vi "BRig_RT__Case_Exp__State_WrongOrTimeout_Pre.vi"(6 "input_dataExp":u16[](array[numeric]), 8 "input_dataTrial":u16[][](array[numeric]), 9 "input_dataBlock":u16[][](array[numeric]), 10 "input_WorTO":bool, 11 "input_dataCurrent":u16[](array[numeric])) -> (0 "output_dataTrial":u16[][](array[numeric]), 1 "output_dataBlock":u16[][](array[numeric]), 2 "output_T2R_or_BTPR":u16, 3 "output_dataCurrent":u16[](array[numeric]), 5 "output_T2R":bool, 7 "output_BTPR":bool)   [LabVIEW 2014]
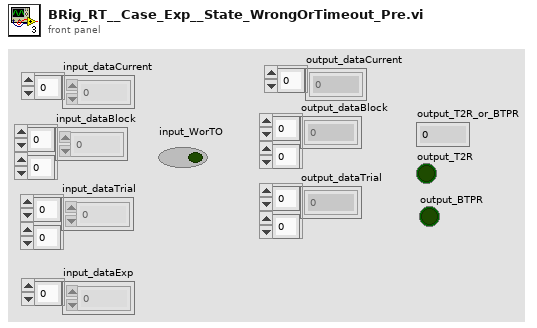
[diagram p1: front panel]
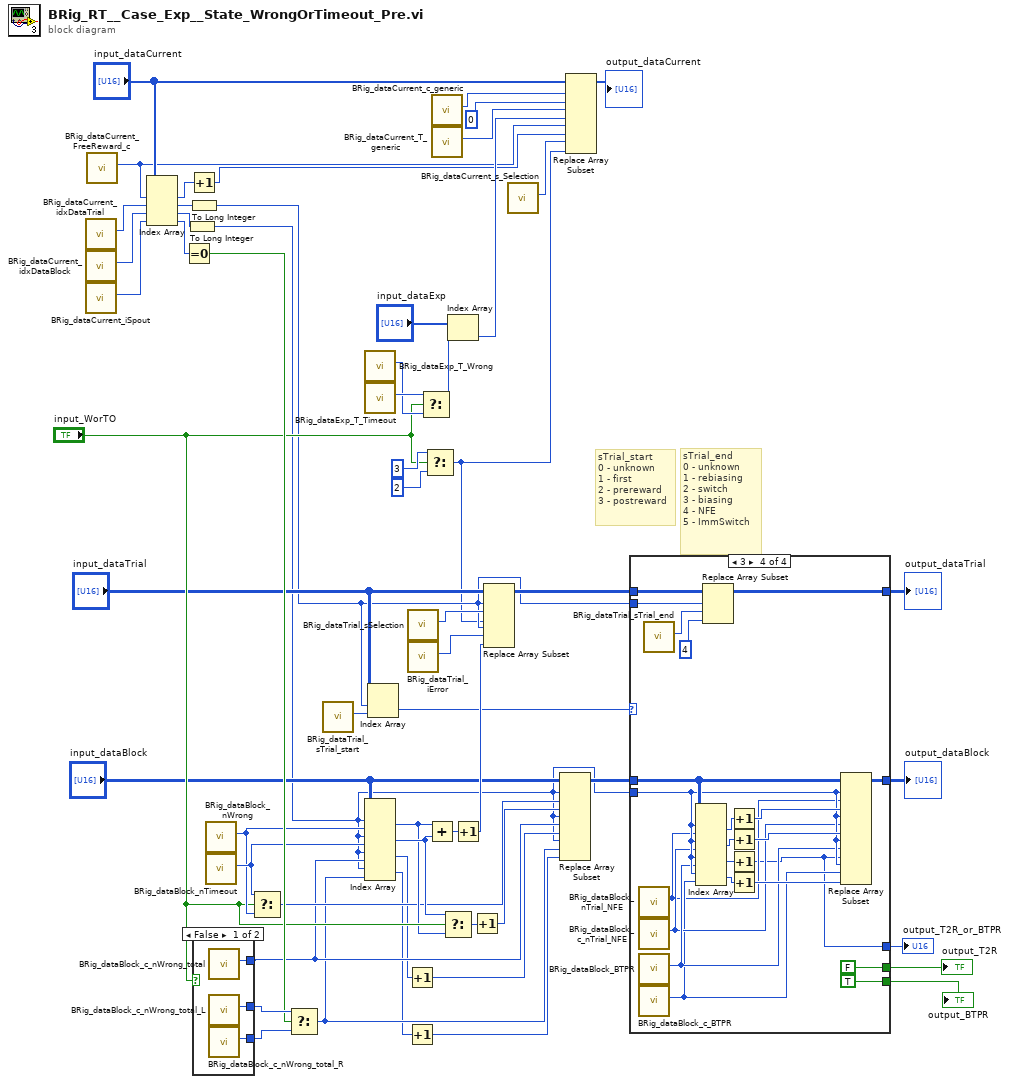
[diagram p0: block diagram]
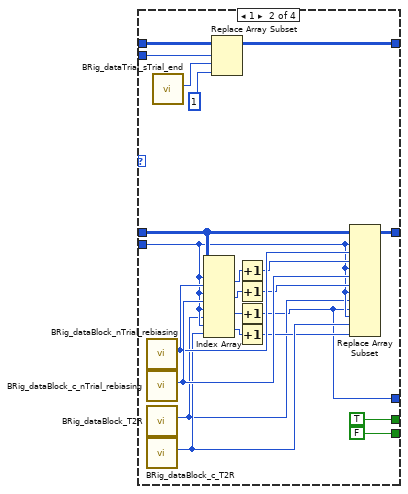
[diagram p3: hidden frame]
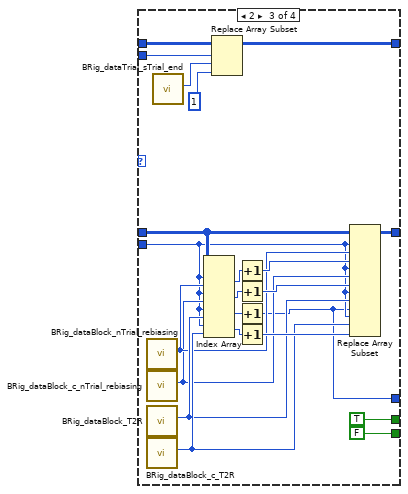
[diagram p4: hidden frame]
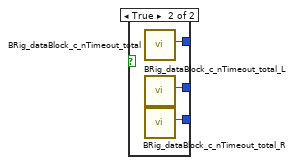
[diagram p5: hidden frame]
diagram:
  # "sTrial_end\n0 - unknown\n1 - rebiasing\n2 - switch\n3 - biasing\n4 - NFE\n5 - ImmSwitch"
  # "sTrial_start\n0 - unknown\n1 - first\n2 - prereward\n3 - postreward"
  n1 = call "BRig_dataCurrent_idxDataTrial.vi"() -> ("output_idxDataTrial"=w53:i32)  [unwired: 11 in]
  n2 = call "BRig_dataCurrent_idxDataBlock.vi"() -> ("output_idxDataBlock"=w51:i32)  [unwired: 11 in]
  n3 = call "BRig_dataCurrent_iSpout.vi"() -> ("output_iSpout"=w49:i32)  [unwired: 11 in]
  n4 = call "BRig_dataCurrent_FreeReward_c.vi"() -> ("output_FreeReward_c"=w8:i32)  [unwired: 11 in]
  n5 = Index Array(array="input_dataCurrent", index #1=w8, index #2=w53, index #3=w51, index #4=w49) -> (element #1=w9:u16, element #2=w52:u16, element #3=w50:u16, element #4=w48:u16)
  n6 = Equal To 0?(x=w48) -> (x = 0?=w33:bool)
  n7 = To Long Integer(number=w50) -> (32bit integer=w13:i32)
  n8 = Increment(x=w9) -> (x+1=w7:u16)
  n9 = To Long Integer(number=w52) -> (32bit integer=w5:i32)
  n10 = case shown="False" "input_WorTO" {
    tunnel: [w60 w63] -> w23
    tunnel: [w59 w62] -> w37
    tunnel: [w58 w61] -> w36
    frame False {
      n11 = call "BRig_dataBlock_c_nWrong_total.vi"() -> ("output_c_nWrong_total"=w60:i32)  [unwired: 11 in]
      n12 = call "BRig_dataBlock_c_nWrong_total_L.vi"() -> ("output_c_nWrong_total_L"=w59:i32)  [unwired: 11 in]
      n13 = call "BRig_dataBlock_c_nWrong_total_R.vi"() -> ("output_c_nWrong_total_R"=w58:i32)  [unwired: 11 in]
    }
    frame True {
      n14 = call "BRig_dataBlock_c_nTimeout_total.vi"() -> ("output_c_nTimeout_total"=w63:i32)  [unwired: 11 in]
      n15 = call "BRig_dataBlock_c_nTimeout_total_L.vi"() -> ("output_c_nTimeout_total_L"=w62:i32)  [unwired: 11 in]
      n16 = call "BRig_dataBlock_c_nTimeout_total_R.vi"() -> ("output_c_nTimeout_total_R"=w61:i32)  [unwired: 11 in]
    }
  }
  n17 = call "BRig_dataBlock_nWrong.vi"() -> ("output_nWrong"=w31:i32)  [unwired: 11 in]
  n18 = call "BRig_dataBlock_nTimeout.vi"() -> ("output_nTimeout"=w32:i32)  [unwired: 11 in]
  n19 = Select(t=w32, s="input_WorTO", f=w31) -> (s? t:f=w25:i32)
  n20 = Select(t=w37, s=w33, f=w36) -> (s? t:f=w22:i32)
  n21 = call "BRig_dataTrial_sTrial_start.vi"() -> ("output_sTrial_start"=w17:i32)  [unwired: 11 in]
  n22 = call "BRig_dataExp_T_Wrong.vi"() -> ("output_T_Wrong"=w43:i32)  [unwired: 11 in]
  n23 = call "BRig_dataExp_T_Timeout.vi"() -> ("output_T_Timeout"=w44:i32)  [unwired: 11 in]
  n24 = Index Array(array="input_dataBlock", index (row) #1=w13, index (col) #1=w31, index (row) #2=w13, index (col) #2=w32, index (row) #3=w13, index (col) #3=w23, index (row) #4=w13, index (col) #4=w22) -> (element #1=w28:u16, element #2=w29:u16, element #3=w21:u16, element #4=w20:u16)
  n25 = Index Array(array="input_dataTrial", index (row)=w5, index (col)=w17) -> (element=w12:u16)
  n26 = Increment(x=w21) -> (x+1=w19:u16)
  n27 = Increment(x=w20) -> (x+1=w18:u16)
  n28 = call "BRig_dataTrial_sSelection.vi"() -> ("output_sSelection"=w39:i32)  [unwired: 11 in]
  n29 = call "BRig_dataTrial_iError.vi"() -> ("output_iError"=w38:i32)  [unwired: 11 in]
  n30 = Select(t=w44, s="input_WorTO", f=w43) -> (s? t:f=w45:i32)
  n31 = Select(t=u16 3 ("new element/subarray"), s="input_WorTO", f=u16 2 ("new element/subarray")) -> (s? t:f=w4:u16)
  n32 = Add(x=w28, y=w29) -> (x+y=w35:u16)
  n33 = call "BRig_dataCurrent_c_generic.vi"() -> ("output_count_generic"=w56:i32)  [unwired: 11 in]
  n34 = call "BRig_dataCurrent_T_generic.vi"() -> ("output_T_generic"=w55:i32)  [unwired: 11 in]
  n35 = Select(t=w29, s="input_WorTO", f=w28) -> (s? t:f=w27:u16)
  n36 = Index Array(array="input_dataExp", index=w45) -> (element=w42:u16)
  n37 = Increment(x=w35) -> (x+1=w34:u16)
  n38 = Increment(x=w27) -> (x+1=w24:u16)
  n39 = Replace Array Subset(array="input_dataTrial", new element #1=w4, index (row) #1=w5, index (col) #1=w39, new element #2=w34, index (row) #2=w5, index (col) #2=w38) -> (w15:u16[][])
  n40 = call "BRig_dataCurrent_s_Selection.vi"() -> ("output_s_Selection"=w6:i32)  [unwired: 11 in]
  n41 = Replace Array Subset(array="input_dataBlock", new element #1=w24, index (row) #1=w13, index (col) #1=w25, new element #2=w19, index (row) #2=w13, index (col) #2=w23, new element #3=w18, index (row) #3=w13, index (col) #3=w22) -> (w14:u16[][])
  n42 = Replace Array Subset(array="input_dataCurrent", new element #1=u16 0 ("new element/subarray"), index #1=w56, new element #2=w42, index #2=w55, new element #3=w7, index #3=w8, new element #4=w4, index #4=w6) -> (→"output_dataCurrent":u16[])
  n43 = case shown="3" w12 {
    tunnel: w15 -> [w65 w87 w109 w131]
    tunnel: w5 -> [_ w85 w107 w129]
    tunnel: [w65 w86 w108 w130] -> w10
    tunnel: w14 -> [w64 w76 w93 w119]
    tunnel: [w64 w75 w91 w117] -> w11
    tunnel: w13 -> [_ w72 w92 w118]
    tunnel: [_ w66 w90 w110] -> w3
    tunnel: [_ TRUE TRUE FALSE] -> w2
    tunnel: [_ FALSE FALSE TRUE] -> w1
    frame 0, Default {
    }
    frame 1 {
      n44 = call "BRig_dataBlock_nTrial_rebiasing.vi"() -> ("output_nTrial_rebiasing"=w81:i32)  [unwired: 11 in]
      n45 = call "BRig_dataBlock_c_nTrial_rebiasing.vi"() -> ("output_c_nTrial_rebiasing"=w82:i32)  [unwired: 11 in]
      n46 = call "BRig_dataBlock_T2R.vi"() -> ("output_T2R"=w69:i32)  [unwired: 11 in]
      n47 = call "BRig_dataBlock_c_T2R.vi"() -> ("output_c_T2R"=w71:i32)  [unwired: 11 in]
      n48 = call "BRig_dataTrial_sTrial_end.vi"() -> ("output_sTrial_end"=w84:i32)  [unwired: 11 in]
      n49 = Index Array(array=w76, index (row) #1=w72, index (col) #1=w81, index (row) #2=w72, index (col) #2=w82, index (row) #3=w72, index (col) #3=w69, index (row) #4=w72, index (col) #4=w71) -> (element #1=w80:u16, element #2=w78:u16, element #3=w74:u16, element #4=w73:u16)
      n50 = Replace Array Subset(array=w87, new element=u16 1 ("new element/subarray"), index (row)=w85, index (col)=w84) -> (w86:u16[][])
      n51 = Increment(x=w80) -> (x+1=w79:u16)
      n52 = Increment(x=w78) -> (x+1=w77:u16)
      n53 = Increment(x=w74) -> (x+1=w66:u16)
      n54 = Increment(x=w73) -> (x+1=w70:u16)
      n55 = Replace Array Subset(array=w76, new element #1=w79, index (row) #1=w72, index (col) #1=w81, new element #2=w77, index (row) #2=w72, index (col) #2=w82, new element #3=w66, index (row) #3=w72, index (col) #3=w69, new element #4=w70, index (row) #4=w72, index (col) #4=w71) -> (w75:u16[][])
    }
    frame 2 {
      n56 = call "BRig_dataBlock_nTrial_rebiasing.vi"() -> ("output_nTrial_rebiasing"=w95:i32)  [unwired: 11 in]
      n57 = call "BRig_dataBlock_c_nTrial_rebiasing.vi"() -> ("output_c_nTrial_rebiasing"=w94:i32)  [unwired: 11 in]
      n58 = call "BRig_dataBlock_T2R.vi"() -> ("output_T2R"=w102:i32)  [unwired: 11 in]
      n59 = call "BRig_dataBlock_c_T2R.vi"() -> ("output_c_T2R"=w103:i32)  [unwired: 11 in]
      n60 = call "BRig_dataTrial_sTrial_end.vi"() -> ("output_sTrial_end"=w106:i32)  [unwired: 11 in]
      n61 = Index Array(array=w93, index (row) #1=w92, index (col) #1=w95, index (row) #2=w92, index (col) #2=w94, index (row) #3=w92, index (col) #3=w102, index (row) #4=w92, index (col) #4=w103) -> (element #1=w96:u16, element #2=w98:u16, element #3=w100:u16, element #4=w101:u16)
      n62 = Replace Array Subset(array=w109, new element=u16 1 ("new element/subarray"), index (row)=w107, index (col)=w106) -> (w108:u16[][])
      n63 = Increment(x=w96) -> (x+1=w97:u16)
      n64 = Increment(x=w98) -> (x+1=w99:u16)
      n65 = Increment(x=w100) -> (x+1=w90:u16)
      n66 = Increment(x=w101) -> (x+1=w104:u16)
      n67 = Replace Array Subset(array=w93, new element #1=w97, index (row) #1=w92, index (col) #1=w95, new element #2=w99, index (row) #2=w92, index (col) #2=w94, new element #3=w90, index (row) #3=w92, index (col) #3=w102, new element #4=w104, index (row) #4=w92, index (col) #4=w103) -> (w91:u16[][])
    }
    frame 3 {
      n68 = call "BRig_dataBlock_nTrial_NFE.vi"() -> ("output_nTrial_NFE"=w113:i32)  [unwired: 11 in]
      n69 = call "BRig_dataBlock_c_nTrial_NFE.vi"() -> ("output_c_nTrial_NFE"=w115:i32)  [unwired: 11 in]
      n70 = call "BRig_dataBlock_BTPR.vi"() -> ("output_BTPR"=w116:i32)  [unwired: 11 in]
      n71 = call "BRig_dataBlock_c_BTPR.vi"() -> ("output_c_BTPR"=w114:i32)  [unwired: 11 in]
      n72 = call "BRig_dataTrial_sTrial_end.vi"() -> ("output_sTrial_end"=w128:i32)  [unwired: 11 in]
      n73 = Index Array(array=w119, index (row) #1=w118, index (col) #1=w113, index (row) #2=w118, index (col) #2=w115, index (row) #3=w118, index (col) #3=w116, index (row) #4=w118, index (col) #4=w114) -> (element #1=w120:u16, element #2=w122:u16, element #3=w124:u16, element #4=w125:u16)
      n74 = Replace Array Subset(array=w131, new element=u16 4 ("new element/subarray"), index (row)=w129, index (col)=w128) -> (w130:u16[][])
      n75 = Increment(x=w120) -> (x+1=w121:u16)
      n76 = Increment(x=w122) -> (x+1=w123:u16)
      n77 = Increment(x=w124) -> (x+1=w110:u16)
      n78 = Increment(x=w125) -> (x+1=w126:u16)
      n79 = Replace Array Subset(array=w119, new element #1=w121, index (row) #1=w118, index (col) #1=w113, new element #2=w123, index (row) #2=w118, index (col) #2=w115, new element #3=w110, index (row) #3=w118, index (col) #3=w116, new element #4=w126, index (row) #4=w118, index (col) #4=w114) -> (w117:u16[][])
    }
  }
  "output_dataBlock" <- w11
  "output_dataTrial" <- w10
  "output_T2R_or_BTPR" <- w3
  "output_T2R" <- w2
  "output_BTPR" <- w1
